vi "pcap配置界面.vi"() -> (0 "电子表格字符串":string="pcx_en:15\r\ncmeas_method:CMEAS_DRIFT_ONE\r\ncmeas_rd_sel:CMEAS_RD_10K\r\ncmeas_clk_sel:CMEAS_CLK_20US\r\nseq_time:0\r\ncmeas_fake:CMEAS_FAKE_0\r\ncmeas_avrg:100\r\ncmeas_trig_sel:CMEAS_TRIG_SOFT\r\ncmeas_cycle_time:49\r\ntmeas_cycle_time:TMEAS_CYCTIME_140US\r\ntmeas_trig_sel:TMEAS_TRIG_SOFT\r\ntmeas_avrg:TMEAS_AVRG_0\r\ntmeas_trig_prediv:0\r\ntmeas_fake:TMEAS_FAKE_2\r\ntmeas_method:TMEAS_METHOD_2\r\ndsp_sel:DSP_SRAM\r\ndsp_speed:DSP_FAST\r\ndsp_core:DSP_CORE_NORMAL\r\n")   [LabVIEW 2017]
panel:
  in  "cmeas_cycle_time":u32=1000 caption="CDC周期时间（us）" min=20 max=20480 step=20
  in  "cmeas_avrg":u32=100 caption="电容内部测量平均次数" max=8192
  in  "cmeas_fake":u16(ring) caption="电容假测量次数" items=["CMEAS_FAKE_0", "CMEAS_FAKE_1", "CMEAS_FAKE_2", "CMEAS_FAKE_3", "CMEAS_FAKE_4"]
  in  "cmeas_rd_sel":u16(ring) caption="放电电阻阻值" items=["CMEAS_RD_10K", "CMEAS_RD_30K", "CMEAS_RD_90K", "CMEAS_RD_180K"]
  in  "应用按钮":bool
  out "数组－字符串":string[][](array[string])=[["pcx_en", "cmeas_method", "cmeas_rd_sel", "cmeas_clk_sel", "seq_time", "cmeas_fake", "cmeas_avrg", "cmeas_trig_sel", "cmeas_cycle_time", "tmeas_cycle_time", "tmeas_trig_sel", "tmeas_avrg", "tmeas_trig_prediv", "tmeas_fake", "tmeas_method", "dsp_sel", "dsp_speed", "dsp_core"], ["15", "CMEAS_DRIFT_ONE", "CMEAS_RD_10K", "CMEAS_CLK_20US", "0", "CMEAS_FAKE_0", "100", "CMEAS_TRIG_SOFT", "49", "TMEAS_CYCTIME_140US", "TMEAS_TRIG_SOFT", "TMEAS_AVRG_0", "0", "TMEAS_FAKE_2", "TMEAS_METHOD_2", "DSP_SRAM", "DSP_FAST", "DSP_CORE_NORMAL"]]
  in  "读取配置文件":path=path "D:/资料/临时工作区/大作业 上位机/pcap_param.ini"
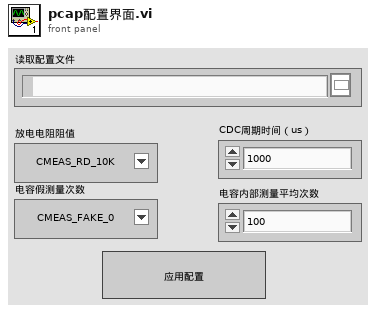
[diagram p1: front panel]
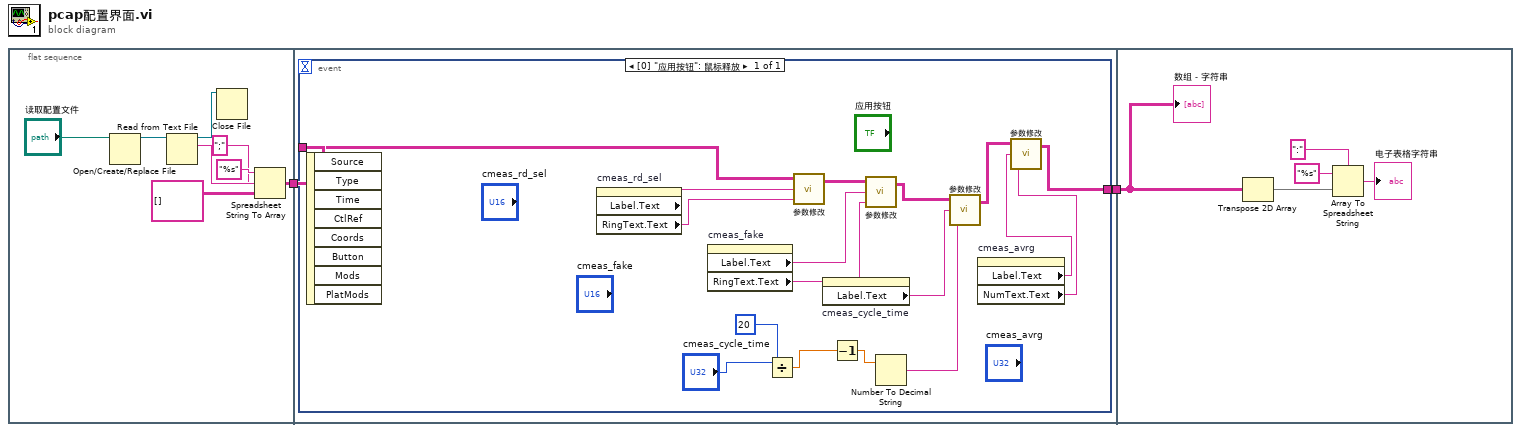
[diagram p0: block diagram]
diagram:
  n1 = flat-sequence {
    tunnel: [w4] -> w2
    tunnel: w2 -> [w12]
    tunnel: [w11] -> w1
    tunnel: w1 -> [w34]
    frame #0 {
      n2 = Open/Create/Replace File(file path (use dialog)="读取配置文件") -> (refnum out=w9:refnum<file>)  [unwired: 5 in, 2 out]
      n3 = Read from Text File(file (use dialog)=w9) -> (refnum out=w3:refnum<file>, text=w8:string)  [unwired: 3 in, 2 out]
      n4 = Close File(refnum=w3) -> ()  [unwired: 1 in, 2 out]
      n5 = Spreadsheet String To Array(delimiter (Tab)=";" ("分隔符(Tab)"), format string="%s" ("格式字符串"), spreadsheet string=w8, array type (2D Dbl)=string[][] [] ("数组类型(2D Dbl)")) -> (array=w4:string[][])
    }
    frame #1 {
      n6 = event shown="[0] \"应用按钮\": 鼠标释放" {
        selector: _ -> [_]
        dyn-events: _ -> [_]
        timeout: _ -> [_]
        tunnel: w12 -> [w28]
        tunnel: [w21] -> w11
        event "应用按钮": Mouse Up {
          n7 = event-data() -> ()  [unwired: 1 in, 8 out]
          n8 = property on="cmeas_rd_sel" class="Ring (严格)"() -> ("Label.Text"=w27:string, "RingText.Text"=w26:string)  [unwired: 2 in, 2 out]
          n9 = property on="cmeas_fake" class="Ring (严格)"() -> ("Label.Text"=w25:string, "RingText.Text"=w24:string)  [unwired: 2 in, 2 out]
          n10 = Divide(x="cmeas_cycle_time", y=u32 20) -> (x/y=w14:dbl)
          n11 = call "参数修改.vi"("参数值"=w26, "参数名"=w27, "输入数组"=w28) -> ("输出数组"=w29:string[][])  [unwired: 1 out]
          n12 = property on="cmeas_cycle_time" class="DigNum (严格)"() -> ("Label.Text"=w20:string)  [unwired: 2 in, 2 out]
          n13 = Decrement(x=w14) -> (x-1=w13:dbl)
          n14 = call "参数修改.vi"("参数值"=w24, "参数名"=w25, "输入数组"=w29) -> ("输出数组"=w23:string[][])  [unwired: 1 out]
          n15 = Number To Decimal String(number=w13) -> (decimal integer string=w15:string)  [unwired: 1 in]
          n16 = call "参数修改.vi"("参数值"=w15, "参数名"=w20, "输入数组"=w23) -> ("输出数组"=w22:string[][])  [unwired: 1 out]
          n17 = property on="cmeas_avrg" class="DigNum (严格)"() -> ("Label.Text"=w19:string, "NumText.Text"=w18:string)  [unwired: 2 in, 2 out]
          n18 = call "参数修改.vi"("参数值"=w18, "参数名"=w19, "输入数组"=w22) -> ("输出数组"=w21:string[][])  [unwired: 1 out]
        }
      }
    }
    frame #2 {
      n19 = Transpose 2D Array(2D array=w34) -> (transposed array=w30:string[][])
      n20 = Array To Spreadsheet String(delimiter (Tab)=":" ("分隔符(Tab)"), array=w30, 3:"%s" ("格式字符串")) -> (spreadsheet string=→"电子表格字符串":string)
      "数组－字符串" <- w34
    }
  }
